vi "TagRotatePixelArray.vi"(1 "Pixel Array In":T1[][](array[typedef])) -> (0 "Rotated Pixel Array":T1[][](array[typedef]))   [LabVIEW 2020, in "g_ar_toolkit.feature_detection.lvlib"]
uses:
  g_ar_toolkit.feature_detection.lvlib
  TagPixelType.ctl
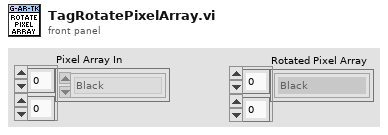
[diagram p1: front panel]
types:
  T1 = typedef "g_ar_toolkit.feature_detection.lvlib/TagPixelType.ctl" = enum8{"Black", "White", "Transparent"}
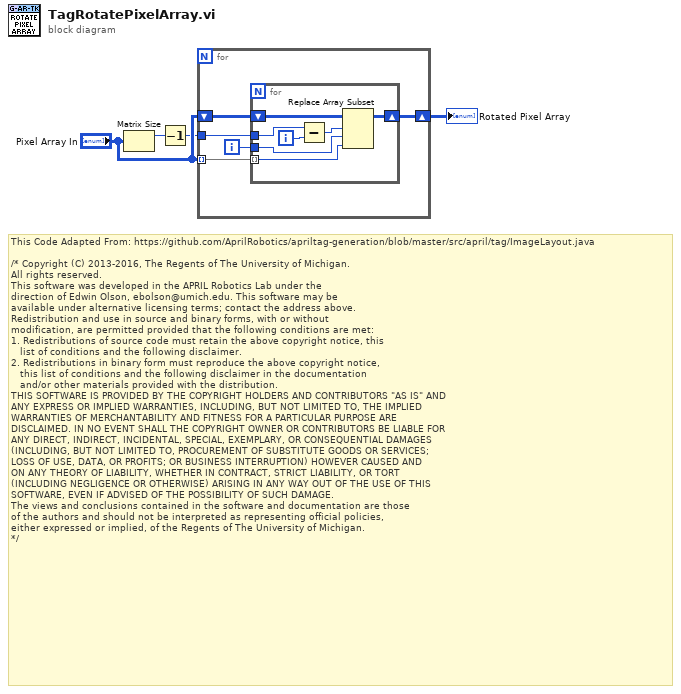
[diagram p0: block diagram]
diagram:
  # "This Code Adapted From: https://github.com/AprilRobotics/apriltag-generation/blob/master/src/april/tag/ImageLayout.java\n\n/* Copyright (C) 2013-2016, The Regents of The University of Michigan.\nAll rights reserved.\nThis software was developed in the APRIL Robotics Lab under the\ndirection of Edwin Olson, ebolson@umich.edu. This software may be\navailable under alternative licensing terms; contact the address above.\nRedistribution and use in source and binary forms, with or without\nmodification, are permitted provided that the following conditions are met:\n1. Redistributions of source code must retain the above copyright notice, this\n   list of conditions and the following disclaimer.\n2. Redistributions in binary form must reproduce the above copyright notice,\n   this list of conditions and the following disclaimer in the documentation\n   and/or other materials provided with the distribution.\nTHIS SOFTWARE IS PROVIDED BY THE COPYRIGHT HOLDERS AND CONTRIBUTORS \"AS IS\" AND\nANY EXPRESS OR IMPLIED WARRANTIES, INCLUDING, BUT NOT LIMITED TO, THE IMPLIED\nWARRANTIES OF MERCHANTABILITY AND FITNESS FOR A PARTICULAR PURPOSE ARE\nDISCLAIMED. IN NO EVENT SHALL THE COPYRIGHT OWNER OR CONTRIBUTORS BE LIABLE FOR\nANY DIRECT, INDIRECT, INCIDENTAL, SPECIAL, EXEMPLARY, OR CONSEQUENTIAL DAMAGES\n(INCLUDING, BUT NOT LIMITED TO, PROCUREMENT OF SUBSTITUTE GOODS OR SERVICES;\nLOSS OF USE, DATA, OR PROFITS; OR BUSINESS INTERRUPTION) HOWEVER CAUSED AND\nON ANY THEORY OF LIABILITY, WHETHER IN CONTRACT, STRICT LIABILITY, OR TORT\n(INCLUDING NEGLIGENCE OR OTHERWISE) ARISING IN ANY WAY OUT OF THE USE OF THIS\nSOFTWARE, EVEN IF ADVISED OF THE POSSIBILITY OF SUCH DAMAGE.\nThe views and conclusions contained in the software and documentation are those\nof the authors and should not be interpreted as representing official policies,\neither expressed or implied, of the Regents of The University of Michigan.\n*/"
  n1 = Matrix Size(0:"Pixel Array In") -> (1:w2:i32)  [unwired: 1 out]
  n2 = Decrement(x=w2) -> (x-1=w1:i32)
  n3 = for {
    tunnel: "Pixel Array In" -> [w9] mode=indexing
    shift-right: [w7] -> w4
    shift-left: "Pixel Array In" -> [w8]
    tunnel: w1 -> [w5]
    i -> [w6]
    n4 = for {
      tunnel: w9 -> [w14] mode=indexing
      shift-right: [w15] -> w7
      shift-left: w8 -> [w16]
      tunnel: w6 -> [w10]
      tunnel: w5 -> [w13]
      i -> [w12]
      n5 = Subtract(x=w13, y=w12) -> (x-y=w11:i32)
      n6 = Replace Array Subset(array=w16, new element=w14, index (row)=w11, index (col)=w10) -> (w15:T1[][])
    }
  }
  "Rotated Pixel Array" <- w4
